vi "Lithographify.vi"(0 "interpolation distance":dbl, 5 "Data In":cluster{string, cluster{"X":dbl, "Y":dbl}[]}, 7 "Direction":u16, 9 "Speed (um/s)":T1 {"Signal Type" items=["Sine Wave", "Triangle Wave", "Square Wave", "Sawtooth Wave"]; "Schedule" items=["Constant", "Ramp", "Fn. Generator", "Formula"]}, 11 "Voltage (V)":T1 {"Signal Type" items=["Sine Wave", "Triangle Wave", "Square Wave", "Sawtooth Wave"]; "Schedule" items=["Constant", "Ramp", "Fn. Generator", "Formula"]}, 13 "Enabled":bool) -> (4 "Lithography Data":T4)   [LabVIEW 2016]
doc: "This VI calculates the lithography data of one pattern and organizes it appropriately."
uses:
  typedefs/Voltage - cluster.ctl
  typedefs/Schedule - enum.ctl
  typedefs/Signal Type - enum.ctl
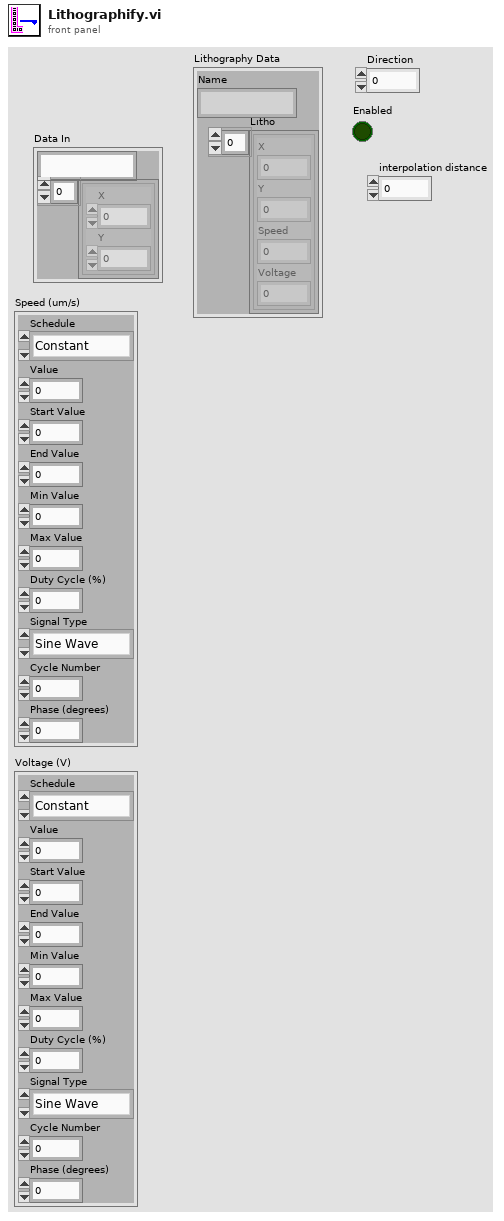
[diagram p1: front panel]
types:
  T1 = typedef "Voltage - cluster.ctl" = cluster{"Schedule":T2, "Value":dbl, "Start Value":dbl, "End Value":dbl, "Min Value":dbl, "Max Value":dbl, "Duty Cycle (%)":dbl, "Signal Type":T3, "Cycle Number":dbl, "Phase (degrees)":dbl}
  T2 = typedef "Schedule - enum.ctl" = u16
  T3 = typedef "Signal Type - enum.ctl" = u16
  T4 = cluster{"Name":string, "Litho":cluster{"X":dbl, "Y":dbl, "Speed":dbl, "Voltage":dbl}[]}
  T5 = cluster{"X":dbl, "Y":dbl, "Speed":dbl, "Voltage":dbl}[]
  T6 = cluster{"X":dbl, "Y":dbl, "Speed":dbl, "Voltage":dbl}
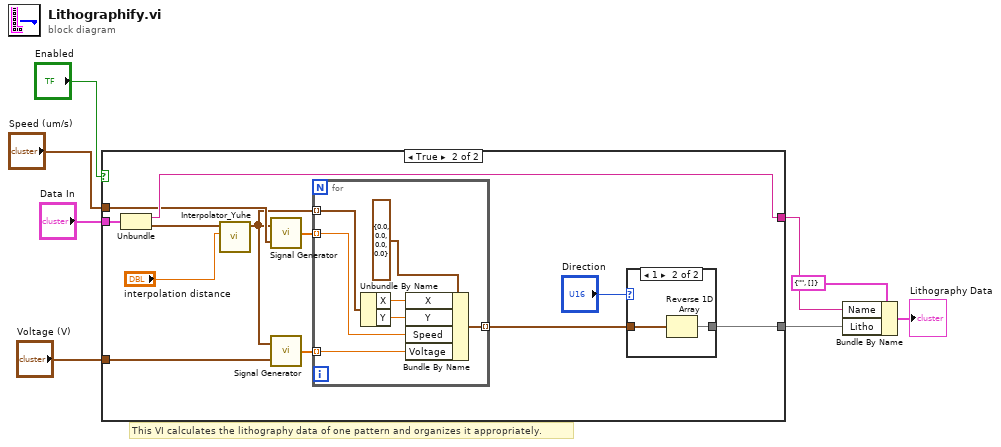
[diagram p0: block diagram]
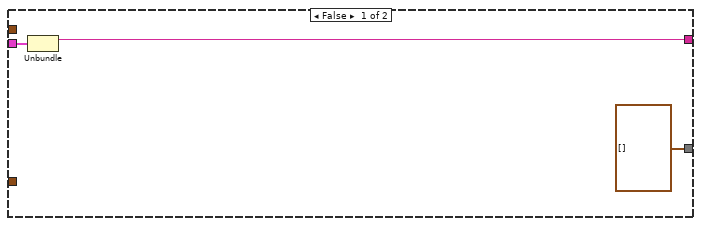
[diagram p2: hidden frame]
diagram:
  # "This VI calculates the lithography data of one pattern and organizes it appropriately."
  n1 = case shown="True" "Enabled" {
    tunnel: [w10 w23] -> w8
    tunnel: "Data In" -> [w11 w22]
    tunnel: "Voltage (V)" -> [_ w19]
    tunnel: "Speed (um/s)" -> [_ w18]
    tunnel: [T5 [] w16] -> w2
    frame False {
      n2 = Unbundle(w11) -> (w10:string)  [unwired: 1 out]
    }
    frame True {
      n3 = Unbundle(w22) -> (w23:string, w14:cluster{"X":dbl, "Y":dbl}[])
      n4 = call "Interpolator_Yuhe.vi"("interpolation distance"="interpolation distance", "Array in"=w14) -> ("Array out"=w12:cluster{"X":dbl, "Y":dbl}[])  [unwired: 9 in]
      n5 = call "Signal Generator.vi"("Signal Properties"=w18, "Points"=w12) -> ("Signal"=w20:dbl[])
      n6 = call "Signal Generator.vi"("Signal Properties"=w19, "Points"=w12) -> ("Signal"=w21:dbl[])
      n7 = for {
        tunnel: w20 -> [w29] mode=indexing
        tunnel: w21 -> [w28] mode=indexing
        tunnel: w12 -> [w31] mode=indexing
        tunnel: [w27] -> w17 mode=indexing
        n8 = Unbundle By Name(w31) -> ("X"=w32:dbl, "Y"=w30:dbl)
        n9 = Bundle By Name(cluster=T6 {"X"=0.0, "Y"=0.0, "Speed"=0.0, "Voltage"=0.0} ("Litho Point"), "X"=w32, "Y"=w30, "Speed"=w29, "Voltage"=w28) -> (w27:T6)
      }
      n10 = case shown="1" "Direction" {
        tunnel: w17 -> [w24 w26]
        tunnel: [w24 w25] -> w16
        frame 0, Default {
        }
        frame 1 {
          n11 = Reverse 1D Array(array=w26) -> (reversed array=w25:T5)
        }
      }
    }
  }
  n12 = Bundle By Name(cluster=T4 {"Name"="", "Litho"=[]} ("Lithography Data"), "Name"=w8, "Litho"=w2) -> (→"Lithography Data":T4)
